vi "create and initialize reentrant instance.vi"(7 "task name":string, 8 "error in":errorcluster, 9 "results reporter":refnum<class "results reporter.lvclass">, 10 "parameters":variant, 11 "function":T1) -> (0 "error out":errorcluster, 3 "call by reference action":refnum<class "call function by reference.lvclass">)   [LabVIEW 2013, in "call function by reference.lvclass"]
uses:
  call function by reference.lvclass
  function definition.ctl
  results reporter/results reporter.lvclass
  call function by reference.lvclass/call function by reference.ctl
  task/task.lvclass
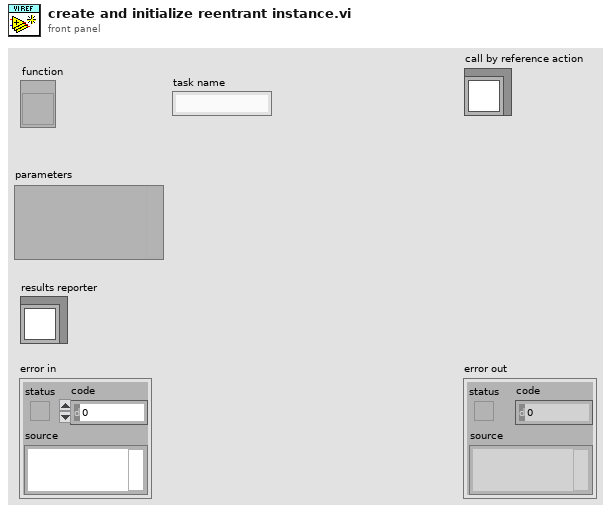
[diagram p1: front panel]
types:
  T1 = typedef "call function by reference.lvclass/function definition.ctl" = refnum<vi>
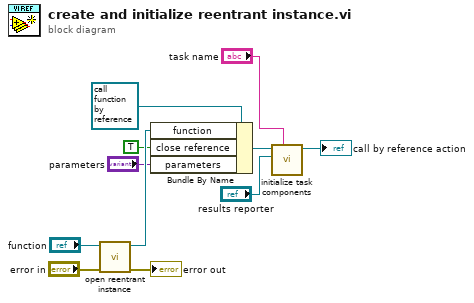
[diagram p0: block diagram]
diagram:
  n1 = call "open reentrant instance.vi"("error in"="error in", "function"="function") -> ("error out"=→"error out":errorcluster, "reentrant instance"=w6:T1)  [unwired: 8 in]
  n2 = Bundle By Name(cluster=refnum<class "call function by reference.lvclass"> refnum ("call by reference action in"), "function"=w6, "close reference"=TRUE, "parameters"="parameters") -> (w9:refnum<class "call function by reference.lvclass">)
  n3 = call "initialize task components.vi"("ID"="task name", "results reporter"="results reporter", "task in"=w9) -> ("task out"=→"call by reference action":refnum<class "call function by reference.lvclass">)  [unwired: 8 in]
